vi "polysol.vi"(8 "y0":dbl, 9 "x0":dbl, 11 "Lane_C_M":dbl[](array[numeric])=[0.8601491478953653, 0.8717844136967624, 0.882947592858927, 0.8936326403234123, 0.9038337699485205, 0.9135454576426009, 0.9227624443554423, 0.9314797389261423, 0.9396926207859084, 0.9473966425143293, 0.9545876322477319, 0.9612616959383189, 0.9674152194628639, 0.9730448705798238, 0.9781476007338057, 0.9827206467064133, 0.9867615321125792, 0.9902680687415704, 0.993238357741943, 0.9956707906498045, 0.9975640502598242, 0.9989171113385246, 0.9997292411794617, 1.0, 0.9997292411794617, 0.9989171113385246, 0.9975640502598242, 0.9956707906498045, 0.993238357741943, 0.9902680687415704, 0.9867615321125792, 0.9827206467064133]) -> (0 "y1":dbl, 1 "x1":dbl, 2 "Y":dbl, 3 "X":dbl)   [LabVIEW 2012]
uses:
  <vilib>/Analysis/polynomials.llb/Polynomial Roots (DBL).vi
  <vilib>/Analysis/NI_AALPro.lvlib
panel:
  out "x-y":u32
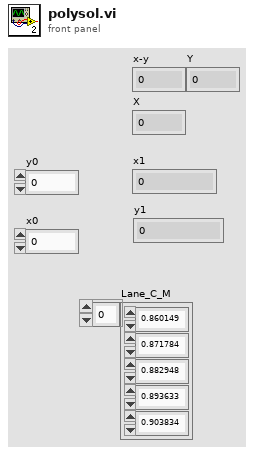
[diagram p1: front panel]
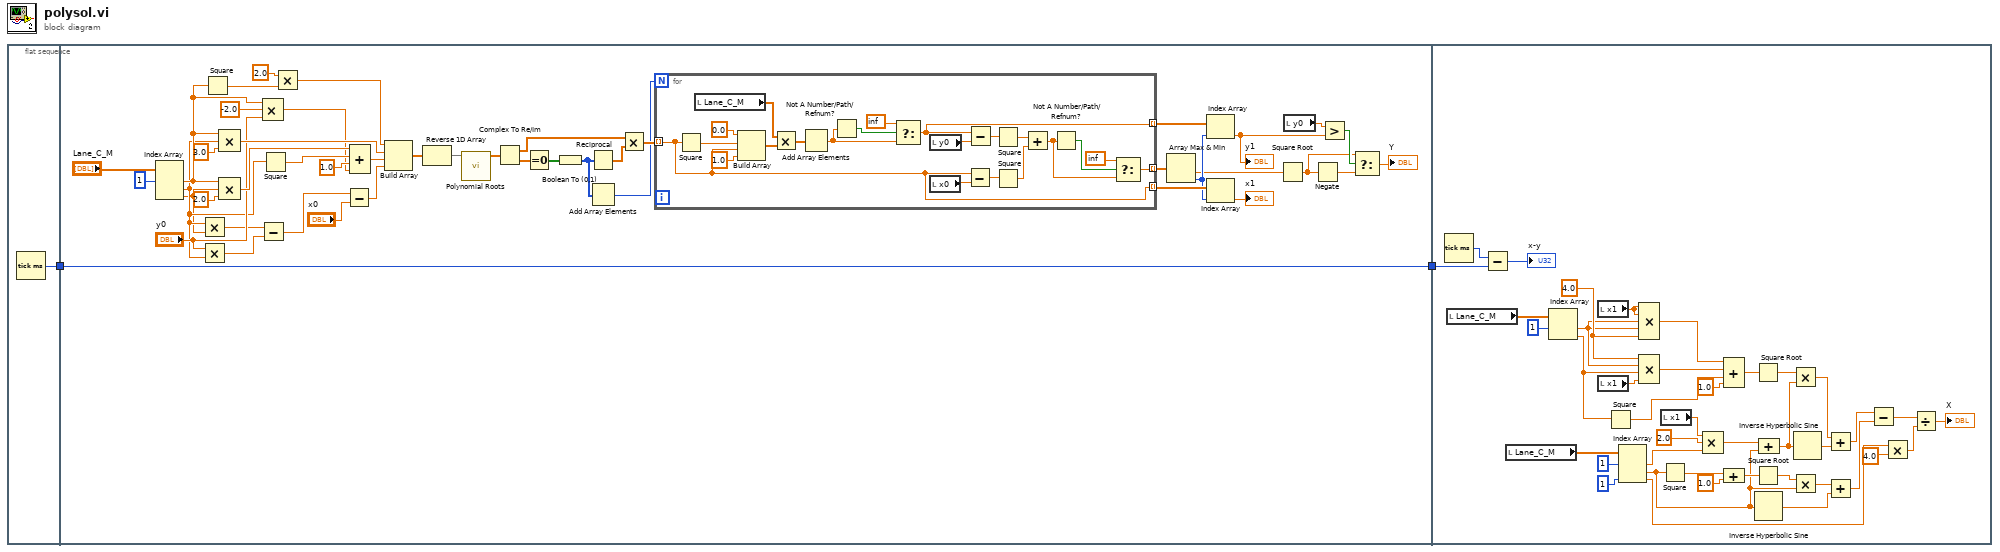
[diagram p0: block diagram]
diagram:
  n1 = flat-sequence {
    tunnel: [w3] -> w1
    tunnel: [w11] -> w2
    tunnel: w1 -> [w11]
    tunnel: w2 -> [w109]
    frame #0 {
      n2 = Tick Count (ms)() -> (millisecond timer value=w3:u32)
    }
    frame #1 {
      n3 = Index Array(array="Lane_C_M", index #1=1 ("index")) -> (element #1=w37:dbl, element #2=w32:dbl, element #3=w31:dbl)  [unwired: 2 in]
      n4 = Multiply(x=w32, y=w31) -> (x*y=w30:dbl)
      n5 = Multiply(x="y0", y=w32) -> (x*y=w29:dbl)
      n6 = Square(x=w37) -> (x^2=w46:dbl)
      n7 = Compound Arithmetic op=MULTIPLY(w37, w32, 3.0 ("value")) -> (w42:dbl)
      n8 = Compound Arithmetic op=MULTIPLY(w37, w31, 2.0 ("value")) -> (w40:dbl)
      n9 = Subtract(x=w30, y=w29) -> (x-y=w28:dbl)
      n10 = Square(x=w32) -> (x^2=w39:dbl)
      n11 = Compound Arithmetic op=MULTIPLY(w37, -2.0 ("value"), "y0") -> (w35:dbl)
      n12 = Multiply(x=2.0, y=w46) -> (x*y=w44:dbl)
      n13 = Subtract(x=w28, y="x0") -> (x-y=w26:dbl)
      n14 = Compound Arithmetic op=ADD(w40, w39, 1.0 ("value"), w35) -> (w34:dbl)
      n15 = Build Array(w44, w42, w34, w26) -> (w25:dbl[])
      n16 = Reverse 1D Array(array=w25) -> (reversed array=w49:dbl[])
      n17 = call-poly <vilib>:"Polynomial Roots.vi"("P(x)"=w49) -> ("Roots"=w24:cdb[])  [unwired: 9 in, 1 out]
      n18 = Complex To Re/Im(x + iy=w24) -> (x=w20:dbl[], y=w23:dbl[])
      n19 = Equal To 0?(x=w23) -> (x = 0?=w22:bool[])
      n20 = Boolean To (0,1)(Boolean=w22) -> (0, 1=w13:i16[])
      n21 = Reciprocal(x=w13) -> (1/x=w21:dbl[])
      n22 = Add Array Elements(numeric array=w13) -> (sum=w12:i16)
      n23 = Multiply(x=w20, y=w21) -> (x*y=w19:dbl[])
      n24 = for {
        N: w12 -> [_]
        tunnel: w19 -> [w50] mode=indexing
        tunnel: [w57] -> w16 mode=indexing
        tunnel: [w54] -> w18 mode=indexing
        tunnel: [w50] -> w17 mode=indexing
        n25 = Square(x=w50) -> (x^2=w69:dbl)
        n26 = local read "Lane_C_M"() -> (w67:dbl[])
        n27 = Build Array(0.0, w69, w50, 1.0 ("element")) -> (w66:dbl[])
        n28 = Multiply(x=w67, y=w66) -> (x*y=w65:dbl[])
        n29 = Add Array Elements(numeric array=w65) -> (sum=w63:dbl)
        n30 = Not A Number/Path/Refnum?(number/path/refnum=w63) -> (NaN/Path/Refnum?=w64:bool)
        n31 = Select(t=inf, s=w64, f=w63) -> (s? t:f=w57:dbl)
        n32 = local read "y0"() -> (w58:dbl)
        n33 = local read "x0"() -> (w61:dbl)
        n34 = Subtract(x=w50, y=w61) -> (x-y=w60:dbl)
        n35 = Subtract(x=w57, y=w58) -> (x-y=w59:dbl)
        n36 = Square(x=w59) -> (x^2=w52:dbl)
        n37 = Square(x=w60) -> (x^2=w51:dbl)
        n38 = Add(x=w52, y=w51) -> (x+y=w53:dbl)
        n39 = Not A Number/Path/Refnum?(number/path/refnum=w53) -> (NaN/Path/Refnum?=w55:bool)
        n40 = Select(t=inf, s=w55, f=w53) -> (s? t:f=w54:dbl)
      }
      n41 = Array Max & Min(array=w18) -> (min value=w10:dbl, min index (indices)=w15:i32)  [unwired: 2 out]
      n42 = Index Array(array=w16, index=w15) -> (element=w8:dbl)
      "y1" <- w8
      n43 = Index Array(array=w17, index=w15) -> (element=→"x1":dbl)
      n44 = Square Root(x=w10) -> (sqrt(x)=w6:dbl)
      n45 = local read "y0"() -> (w9:dbl)
      n46 = Negate(x=w6) -> (-x=w5:dbl)
      n47 = Greater?(x=w9, y=w8) -> (0:w7:bool)
      n48 = Select(t=w6, s=w7, f=w5) -> (s? t:f=→"Y":dbl)
    }
    frame #2 {
      w103 = 4.0 ("value")
      n49 = Tick Count (ms)() -> (millisecond timer value=w110:u32)
      n50 = local read "Lane_C_M"() -> (w107:dbl[])
      n51 = Subtract(x=w110, y=w109) -> (x-y=→"x-y":u32)
      n52 = local read "Lane_C_M"() -> (w94:dbl[])
      n53 = Index Array(array=w107, index #1=1 ("index")) -> (element #1=w102:dbl, element #2=w99:dbl)  [unwired: 1 in]
      n54 = local read "x1"() -> (w105:dbl)
      n55 = local read "x1"() -> (w101:dbl)
      n56 = Square(x=w99) -> (x^2=w98:dbl)
      n57 = Index Array(array=w94, index #1=1 ("index"), index #3=1 ("index")) -> (element #1=w93:dbl, element #2=w76:dbl, element #3=w74:dbl)  [unwired: 1 in]
      n58 = Compound Arithmetic op=MULTIPLY(w105, w105, w102, w102, w103) -> (w104:dbl)
      n59 = Compound Arithmetic op=MULTIPLY(w103, w102, w99, w101) -> (w100:dbl)
      n60 = local read "x1"() -> (w91:dbl)
      n61 = Square(x=w76) -> (x^2=w80:dbl)
      n62 = Compound Arithmetic op=MULTIPLY(w91, 2.0 ("value"), w93) -> (w90:dbl)
      n63 = Compound Arithmetic op=ADD(w104, w100, w98, 1.0 ("value")) -> (w96:dbl)
      n64 = Compound Arithmetic op=ADD(w80, 1.0 ("value")) -> (w82:dbl)
      n65 = Square Root(x=w96) -> (sqrt(x)=w89:dbl)
      n66 = Square Root(x=w82) -> (sqrt(x)=w83:dbl)
      n67 = Inverse Hyperbolic Sine(1:w76) -> (0:w85:dbl)
      n68 = Compound Arithmetic op=ADD(w90, w76) -> (w88:dbl)
      n69 = Multiply(x=w89, y=w88) -> (x*y=w87:dbl)
      n70 = Multiply(x=w83, y=w76) -> (x*y=w84:dbl)
      n71 = Inverse Hyperbolic Sine(1:w88) -> (0:w86:dbl)
      n72 = Add(x=w87, y=w86) -> (x+y=w79:dbl)
      n73 = Add(x=w84, y=w85) -> (x+y=w78:dbl)
      n74 = Subtract(x=w79, y=w78) -> (x-y=w77:dbl)
      n75 = Multiply(x=w74, y=4.0) -> (x*y=w72:dbl)
      n76 = Divide(x=w77, y=w72) -> (x/y=→"X":dbl)
    }
  }
